vi "Exemple_Preprocessing_StandardScaler.vi"() -> ()   [LabVIEW 2020]
uses:
  Objet/6 - Datasets Transformation/6.3 - Processing Data/StandardScaler/StandardScaler.lvclass
panel:
  in  "y":string[][](array[string])
  in  "X":string[][](array[string])=[["0", "0"], ["0", "0"], ["1", "1"], ["1", "1"]]
  out "Data":T1
  out "error out":errorcluster
  in  "error in":errorcluster caption="entrée d'erreur"
  in  "StandardScaler":T2={"copy"=TRUE, "with_mean"=TRUE, "with_std"=TRUE}
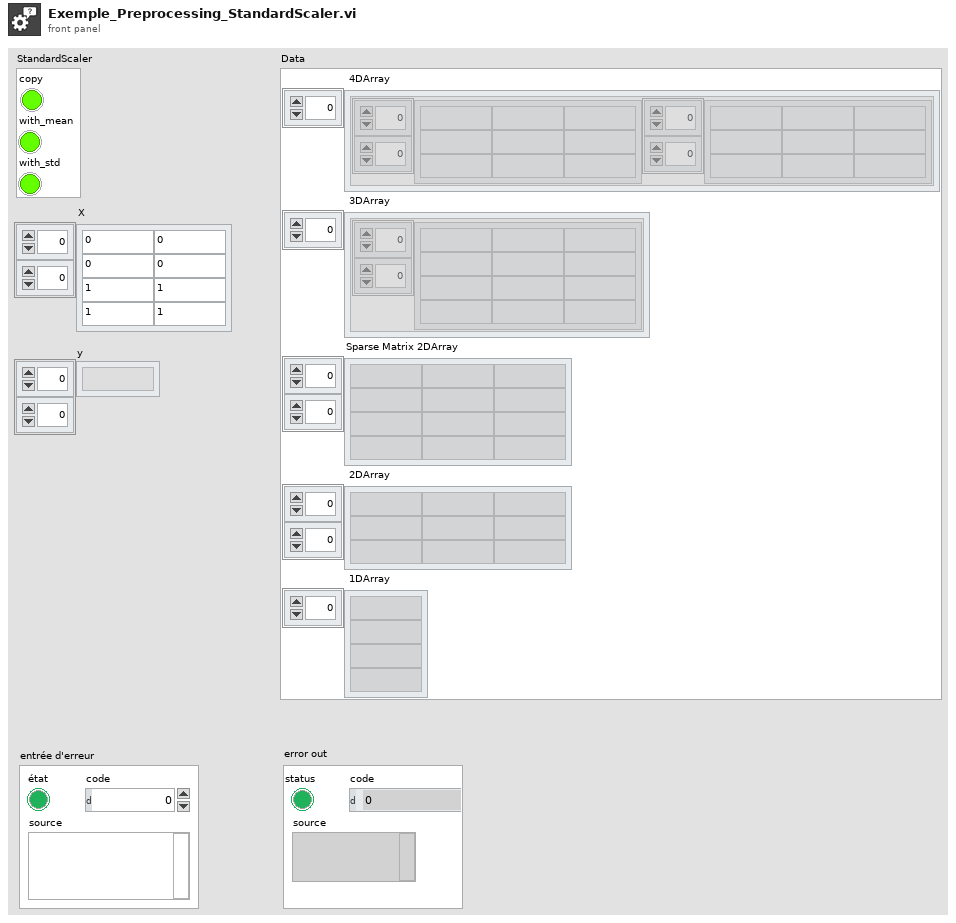
[diagram p1: front panel]
types:
  T1 = cluster{" 4DArray":cluster{"1":string[][], "2":string[][]}[], " 3DArray":cluster{"Tableau":string[][]}[], "Sparse Matrix 2DArray":string[][], " 2DArray":string[][], " 1DArray":string[]}
  T2 = cluster{"copy":bool, "with_mean":bool, "with_std":bool}
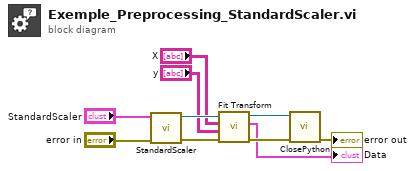
[diagram p0: block diagram]
diagram:
  n1 = call "StandardScaler.vi"("error in (no error)"="error in", "StandardScaler"="StandardScaler") -> ("error out"=w5:errorcluster, "StandardScaler.lvclass"=w8:refnum<class "StandardScaler.lvclass">)  [unwired: 8 in]
  n2 = call-dynamic "Fit Transform.vi"("error in (no error)"=w5, "y"="y", "X"="X", "StandardScaler.lvclass"=w8) -> ("error out"=w4:errorcluster, "Data"=→"Data":T1, "StandardScaler.lvclass"=w3:refnum<class "StandardScaler.lvclass">)  [unwired: 5 in]
  n3 = call-dynamic "ClosePython.vi"("error in (no error)"=w4, "Scikit-learn en entrée"=w3) -> ("error out"=→"error out":errorcluster)  [unwired: 8 in, 1 out]
